vi "Dual_image_synced_snap_p_read_30psi.vi"() -> ()   [LabVIEW 2013]
uses:
  <vilib>/DAQmx/write.llb/DAQmx Write (Analog DBL 1Chan 1Samp).vi
  <vilib>/DAQmx/create/channels.llb/DAQmx Create Channel (AO-Voltage-Basic).vi
  <vilib>/DAQmx/create/channels.llb/DAQmx Create Channel (CO-Pulse Generation-Frequency).vi
  <vilib>/DAQmx/configure/timing.llb/DAQmx Timing (Implicit).vi
  <vilib>/DAQmx/miscellaneous.llb/DAQmx Fill In Error Info.vi
  <vilib>/vision/driver/NI_Vision_Acquisition_Software.lvlib
  <resource>/objmgr/imaqdx.rc
  <resource>/objmgr/daqmx.rc
panel:
  out "Snap Counter":u32
  in  "Snap":bool
  in  "Pressure Frequency (Hz)":dbl=10.0 format="%#_13g"
  in  "im num 2":string
  in  "im time 2":string
  out "im num":string
  out "im time":string
  out "Pressure Reading":cluster{dbl[], dbl[]}(graph)
  in  "Pressure Offset":dbl
  out "Current Pressure (Psi)":dbl format="%#.4g"
  in  "Gain 2":dbl(slide)=575.0 min=350.0 max=1000.0 step=1.0 scale=350.0..1000.0
  in  "VR2":dbl(slide)=65.0 min=0.0 max=255.0 step=1.0 scale=0.0..255.0
  in  "VR1":dbl(slide)=60.0 min=0.0 max=255.0 step=1.0 scale=0.0..255.0
  in  "UB2":dbl(slide)=160.0 min=0.0 max=255.0 step=1.0 scale=0.0..255.0
  in  "UB1":dbl(slide)=165.0 min=0.0 max=255.0 step=1.0 scale=0.0..255.0
  in  "Shutter":dbl(slide)=4095.0 min=0.0 max=4095.0 step=1.0 scale=4.095..4095.0 scale format="%#.0f"
  in  "Brightness":dbl(slide)=100.0 min=0.0 max=255.0 step=1.0 scale=0.0..255.0
  in  "Gain":dbl(slide)=600.0 min=350.0 max=1000.0 step=1.0 scale=350.0..1000.0
  in  "Test Description":string="test"
  in  "Storage Directory":path=path "C:/Users/Regen/Desktop/Users/Ryan Gergely/3D_DIC"
  out "Image 2":T1(plugin-control)
  out "Buffer Number 2":u32
  out "Frame Rate 2":dbl
  in  "Camera Name 2":refnum<k21>="cam2" caption="IMAQdx Session"
  in  "Image Frequency (Hz)":dbl=2.0 format="%.1f"
  out "Actual Duty Cycle":dbl
  out "Actual Frequency":dbl
  in  "Stop":bool
  in  "Start Trigger Mode":bool
  out "Frame Rate 1":dbl
  out "Buffer Number 1":u32
  in  "Camera Name 1":refnum<k21>="cam1" caption="IMAQdx Session"
  out "Image":T1(plugin-control)
  # "Exposure Settings - Both Cameras"
  # "White Balance - Camera1"
  # "White Balance - Camera2"
  # "1) Set Test Description and Storage Directory"
  # "2) Select Cameras"
  # "3) Start VI"
  # "4) Set Frequency and Exposure and White Balance\n(Before Start Trigger)"
  # "5)"
  # "6) Stop When Done"
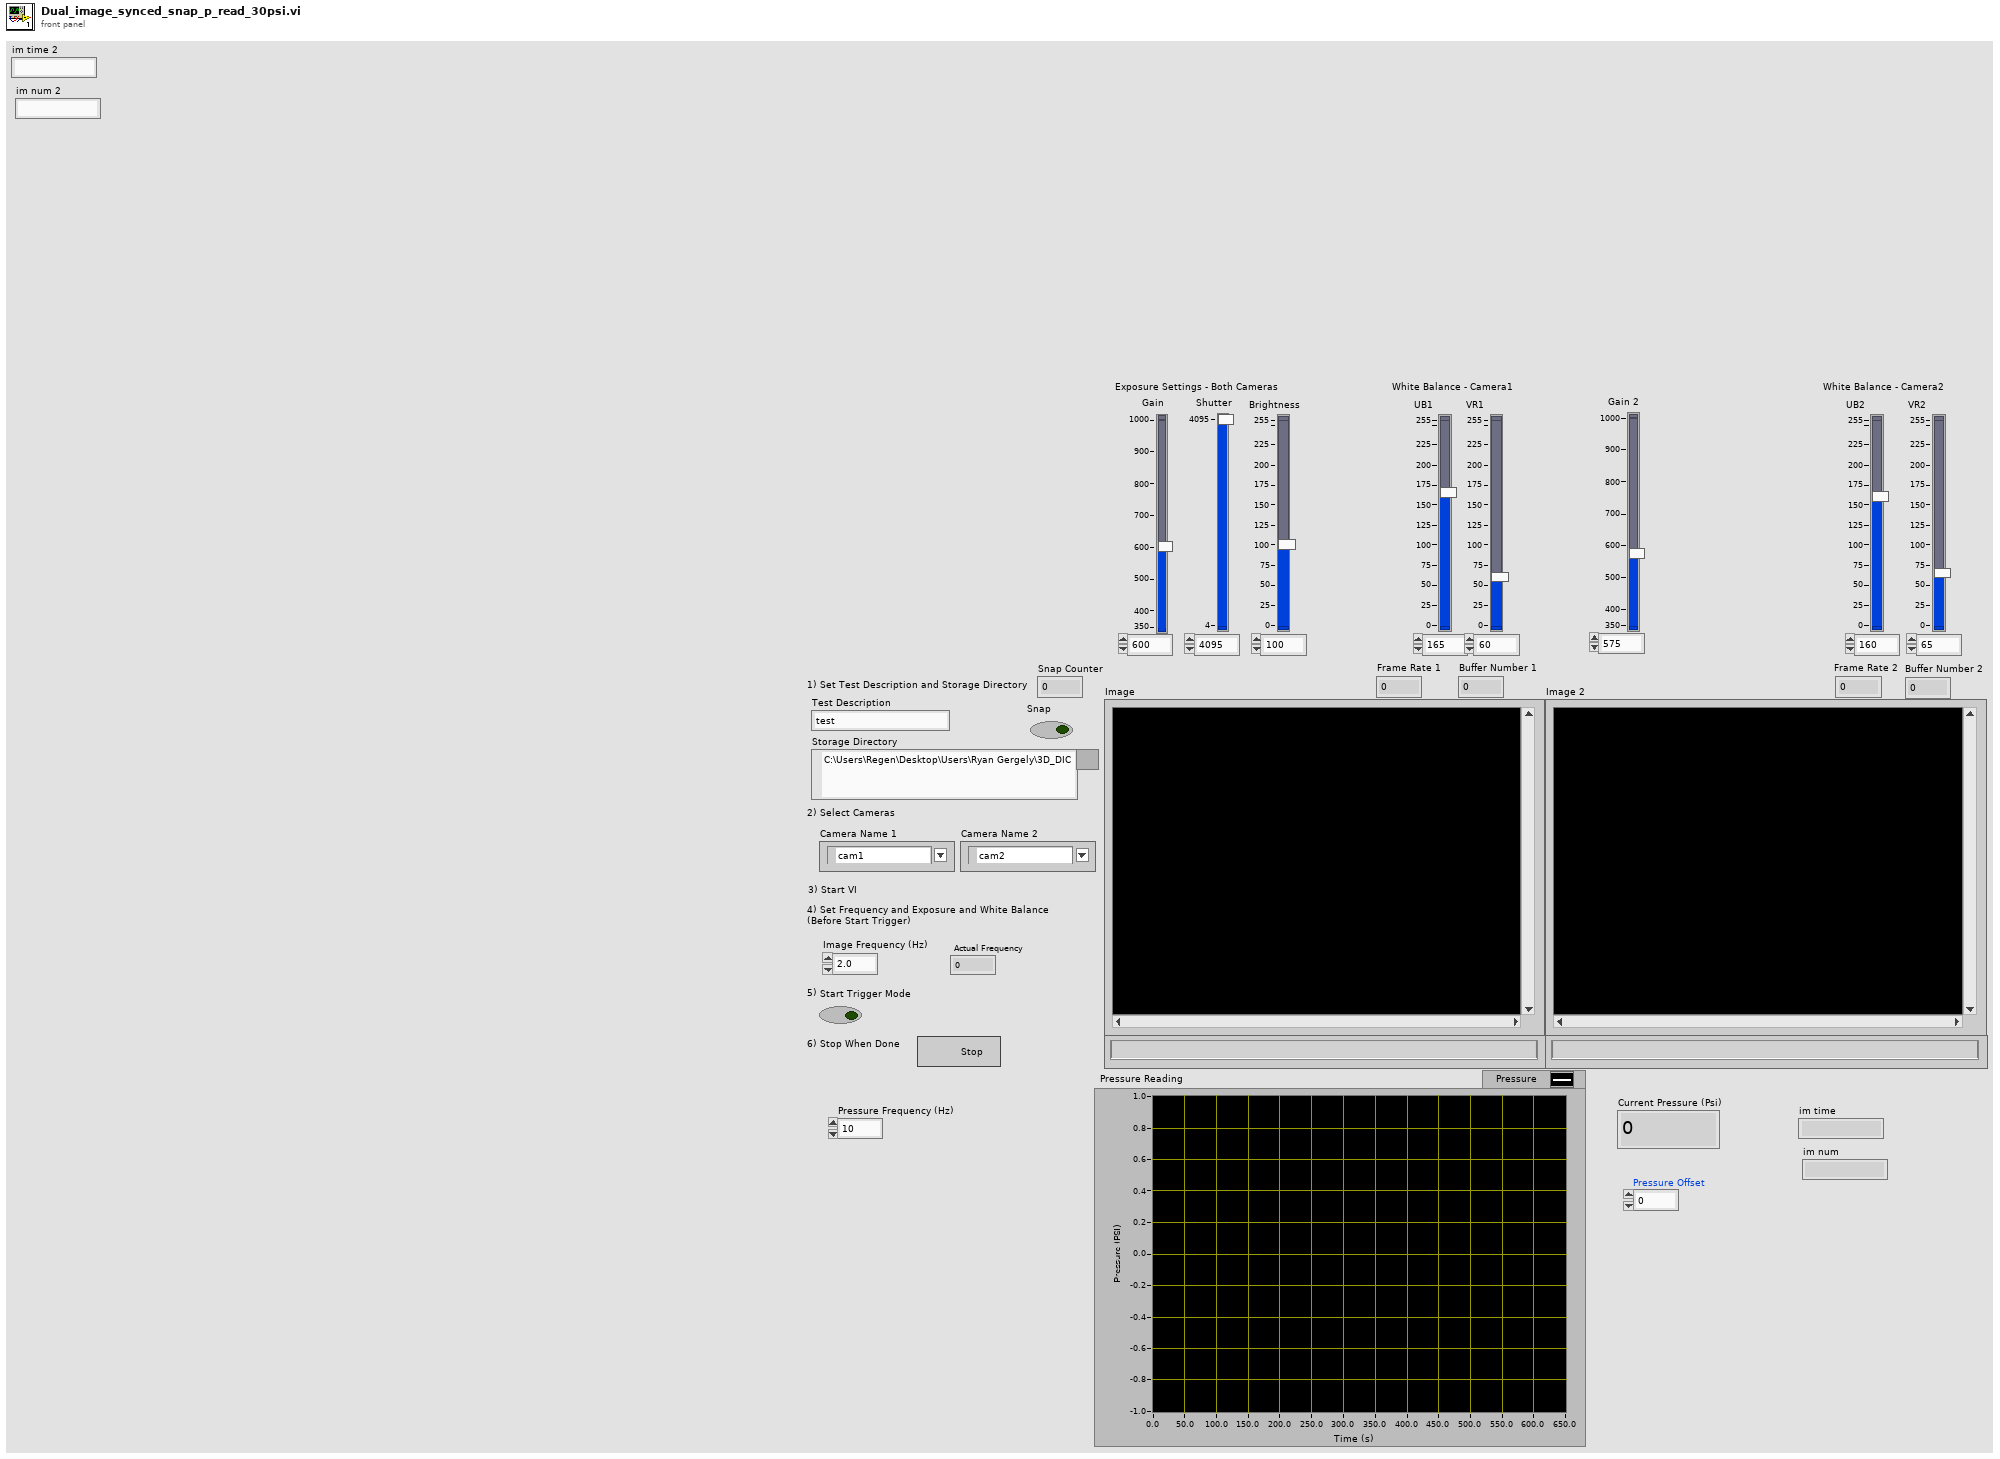
[diagram p1: front panel]
types:
  T1 = typedef "IMAQ Image.ctl" = refnum<image>
  T2 = enum16{"open", "open or create", "create or replace", "create", "open (read only)"}
  T3 = typedef "IMAQdx.ctl" = refnum<k21>
  T4 = enum16{"open", "replace", "create", "open or create", "replace or create", "replace or create with confirmation"}
  T5 = cluster{"Trigger Mode":u32, "Trigger Activation":u32, "Timeout (ms)":u32}
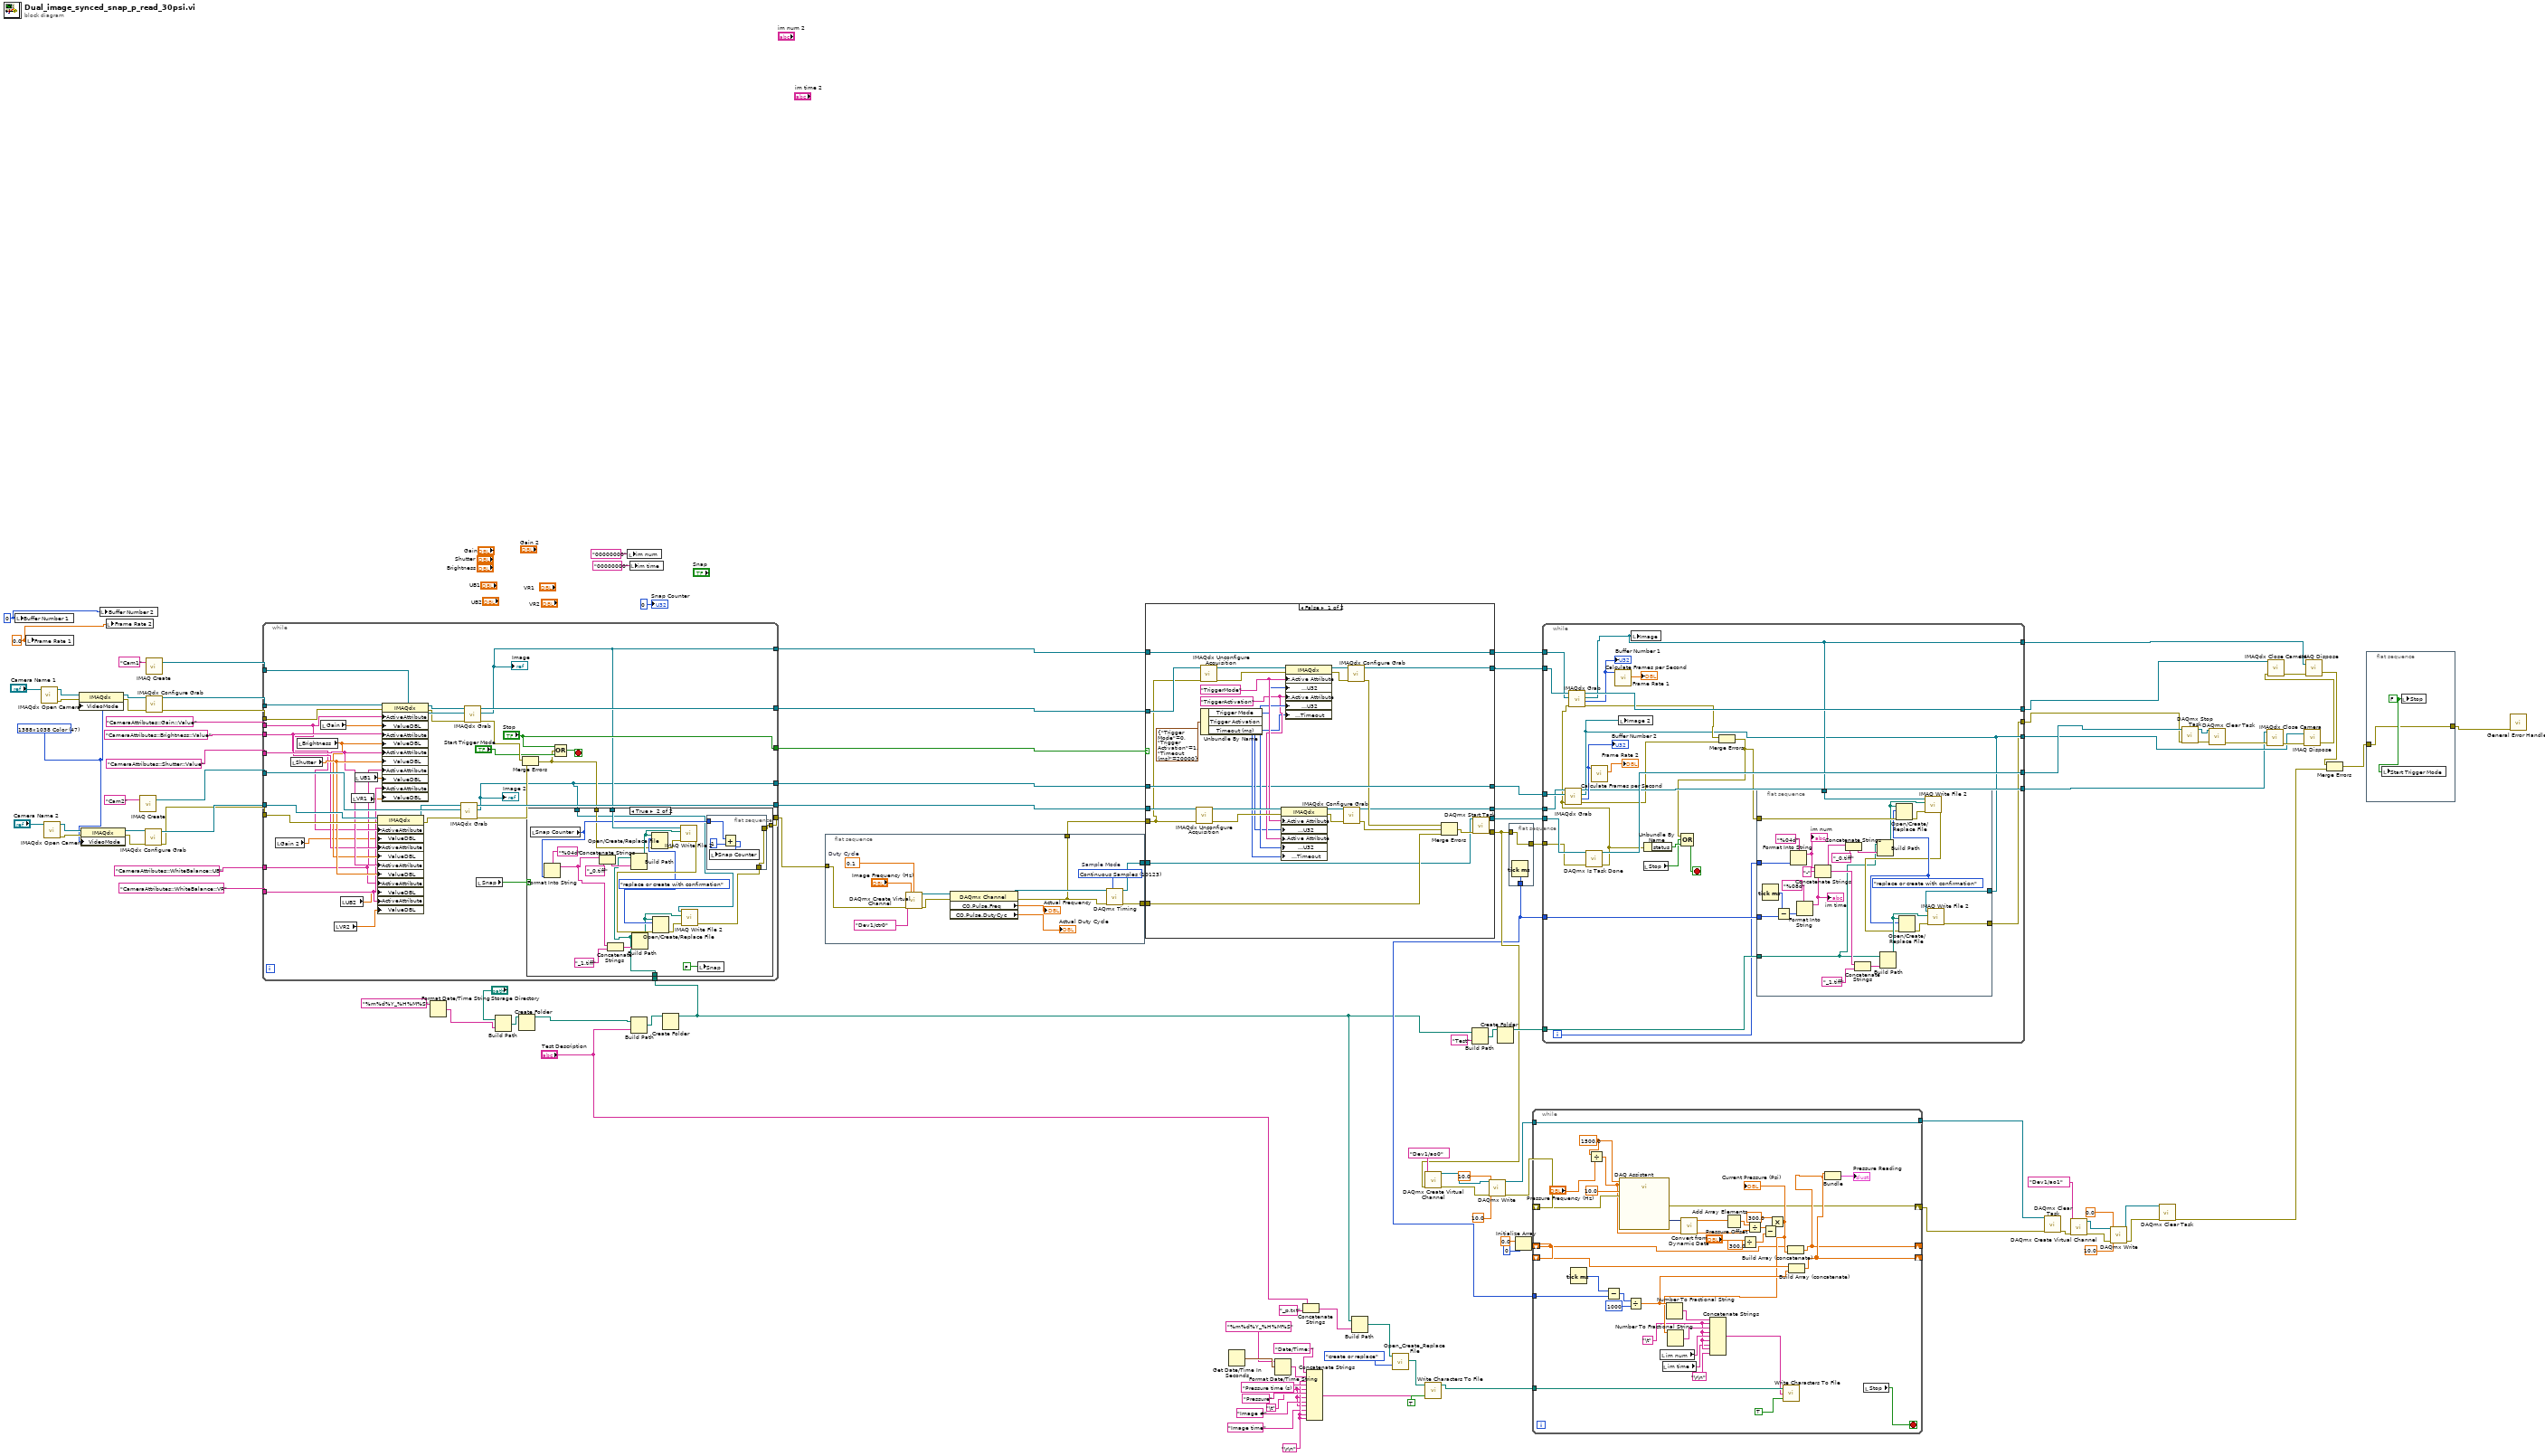
[diagram p0: block diagram]
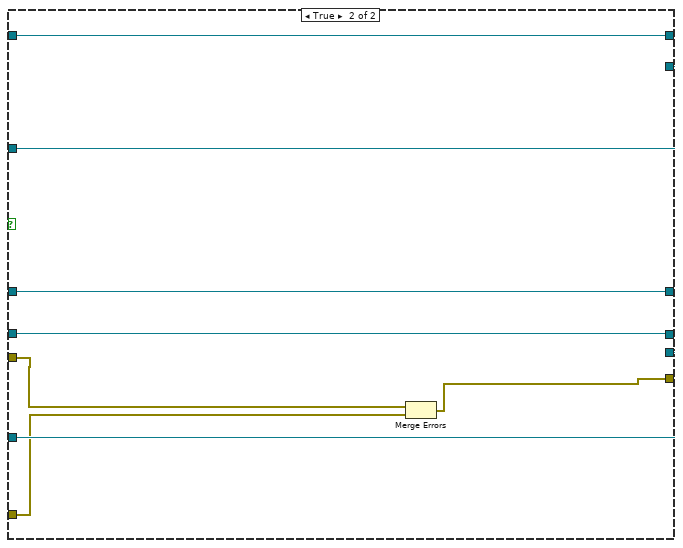
[diagram p2: hidden frame]
diagram:
  w2 = "\t"
  w4 = "\r\n"
  w61 = u32 47 items=["320x240 Color"=4, "640x480 Mono8"=9, "640x480 Mono16"=19, "640x480 Color"=14, "800x600 Mono8"=21, "800x600 Mono16"=27, "800x600 Color"=24, "1024x768 Mono8"=30, "1024x768 Mono16"=36, "1024x768 Color"=33, "1280x960 Mono8"=40, "1280x960 Mono16"=46, "1280x960 Color"=43, "1388x1038 Color"=47, "1388x1038 Mono"=48] ("Video Mode")
  w62 = 0.0 ("Frame Rate 1")
  w63 = u32 0 ("Buffer Number 1")
  n1 = local write "Buffer Number 1"(w63) -> ()
  n2 = local write "Frame Rate 1"(w62) -> ()
  n3 = call <vilib>:"IMAQdx Open Camera.vi"("Session In"="Camera Name 1") -> ("error out"=w69:errorcluster, "Session Out"=w71:T3)  [unwired: 2 in, 7 out]
  n4 = call <vilib>:"IMAQdx Open Camera.vi"("Session In"="Camera Name 2") -> ("error out"=w64:errorcluster, "Session Out"=w65:T3)  [unwired: 2 in, 7 out]
  n5 = property class="IMAQdx"(reference=w71, error in=w69, "VideoMode"=w61) -> (reference out=w70:T3, error out=w68:errorcluster)
  n6 = property class="IMAQdx"(reference=w65, error in=w64, "VideoMode"=w61) -> (reference out=w67:T3, error out=w66:errorcluster)
  n7 = local write "Buffer Number 2"(w63) -> ()
  n8 = local write "Frame Rate 2"(w62) -> ()
  n9 = call "IMAQ Create"("Image Name"="Cam2") -> ("New Image"=w58:T1)  [unwired: 3 in, 2 out]
  n10 = call <vilib>:"IMAQdx Configure Grab.vi"("error in"=w66, "Session In"=w67) -> ("error out"=w91:errorcluster, "Session Out"=w92:T3)  [unwired: 8 out]
  n11 = call "IMAQ Create"("Image Name"="Cam1") -> ("New Image"=w102:T1)  [unwired: 3 in, 2 out]
  n12 = call <vilib>:"IMAQdx Configure Grab.vi"("error in"=w68, "Session In"=w70) -> ("error out"=w100:errorcluster, "Session Out"=w101:T3)  [unwired: 8 out]
  n13 = Format Date/Time String(time format string (%c)="%m%d%Y_%H%M%S") -> (date/time string=w77:string)  [unwired: 2 in]
  n14 = Build Path(base path="Storage Directory", name or relative path=w77) -> (appended path=w79:path)
  n15 = Create Folder(path (use dialog)=w79) -> (created path=w27:path)  [unwired: 2 in, 2 out]
  n16 = local write "im num"("00000000" ("im num 2")) -> ()
  n17 = local write "im time"("00000000" ("im time 2")) -> ()
  n18 = Build Path(base path=w27, name or relative path="Test Description") -> (appended path=w75:path)
  n19 = Create Folder(path (use dialog)=w75) -> (created path=w6:path)  [unwired: 2 in, 2 out]
  n20 = while {
    tunnel: [w147] -> w109
    tunnel: w100 -> [w140]
    tunnel: w101 -> [w142]
    tunnel: w102 -> [w144]
    tunnel: [w116] -> w97
    tunnel: ["Stop"] -> w98
    tunnel: w92 -> [w138]
    tunnel: w91 -> [w137]
    tunnel: [w117] -> w60
    tunnel: [w145] -> w90
    tunnel: [w112] -> w89
    tunnel: w58 -> [w143]
    tunnel: "CameraAttributes::Shutter::Value" ("ActiveAttribute") -> [w133]
    tunnel: "CameraAttributes::Brightness::Value" ("ActiveAttribute") -> [w131]
    tunnel: "CameraAttributes::Gain::Value" ("ActiveAttribute") -> [w129]
    tunnel: "CameraAttributes::WhiteBalance::UB" ("ActiveAttribute") -> [w126]
    tunnel: "CameraAttributes::WhiteBalance::VR" ("ActiveAttribute") -> [w127]
    tunnel: w6 -> [w114]
    stop <- w121 stop-if-true
    n21 = local read "Gain 2"() -> (w122:dbl)
    n22 = local read "Shutter"() -> (w134:dbl)
    n23 = local read "Brightness"() -> (w132:dbl)
    n24 = local read "Gain"() -> (w130:dbl)
    n25 = local read "VR2"() -> (w123:dbl)
    n26 = local read "UB2"() -> (w125:dbl)
    n27 = local read "VR1"() -> (w124:dbl)
    n28 = local read "UB1"() -> (w128:dbl)
    n29 = property class="IMAQdx"(reference=w138, error in=w137, "ActiveAttribute"=w129, "ValueDBL"=w122, "ActiveAttribute"=w131, "ValueDBL"=w132, "ActiveAttribute"=w133, "ValueDBL"=w134, "ActiveAttribute"=w126, "ValueDBL"=w125, "ActiveAttribute"=w127, "ValueDBL"=w123) -> (reference out=w135:T3, error out=w136:errorcluster)
    n30 = property class="IMAQdx"(reference=w142, error in=w140, "ActiveAttribute"=w129, "ValueDBL"=w130, "ActiveAttribute"=w131, "ValueDBL"=w132, "ActiveAttribute"=w133, "ValueDBL"=w134, "ActiveAttribute"=w126, "ValueDBL"=w128, "ActiveAttribute"=w127, "ValueDBL"=w124) -> (reference out=w141:T3, error out=w139:errorcluster)
    n31 = call <vilib>:"IMAQdx Grab.vi"("error in"=w136, "Image In"=w143, "Session In"=w135) -> ("error out"=w118:errorcluster, "Image Out"=w112:T1, "Session Out"=w145:T3)  [unwired: 1 in, 5 out]
    "Image 2" <- w112
    n32 = call <vilib>:"IMAQdx Grab.vi"("error in"=w139, "Image In"=w144, "Session In"=w141) -> ("error out"=w120:errorcluster, "Image Out"=w116:T1, "Session Out"=w147:T3)  [unwired: 1 in, 5 out]
    "Image" <- w116
    n33 = local read "Snap"() -> (w113:bool)
    n34 = Merge Errors(w120, w118) -> (w115:errorcluster)
    n35 = case shown="True" w113 {
      tunnel: [w148 w153] -> w117
      tunnel: w116 -> [_ w157]
      tunnel: w114 -> [_ w151]
      tunnel: w115 -> [w148 w150]
      tunnel: w112 -> [_ w149]
      frame False {
      }
      frame True {
        w160 = T4."replace or create with confirmation" ("operation (0:open)")
        n36 = local read "Snap Counter"() -> (w155:u32)
        n37 = Format Into String(format string="%04d", w155) -> (resulting string=w152:string)  [unwired: 2 in, 1 out]
        n38 = Concatenate Strings(w152, "_0.tiff") -> (w165:string)
        n39 = Concatenate Strings(w152, "_1.tiff") -> (w164:string)
        n40 = Build Path(base path=w151, name or relative path=w165) -> (appended path=w158:path)
        n41 = Build Path(base path=w151, name or relative path=w164) -> (appended path=w159:path)
        n42 = Open/Create/Replace File(file path (use dialog)=w158, error in=w150, operation (0:open)=w160) -> (error out=w161:errorcluster)  [unwired: 3 in, 2 out]
        n43 = call-poly "IMAQ Write File 2"("error in (no error)"=w161, "File Path"=w158, "Image"=w157) -> ("error out"=w163:errorcluster)  [unwired: 7 in, 1 out]
        n44 = Open/Create/Replace File(file path (use dialog)=w159, error in=w163, operation (0:open)=w160) -> (error out=w162:errorcluster)  [unwired: 3 in, 2 out]
        n45 = call-poly "IMAQ Write File 2"("error in (no error)"=w162, "File Path"=w159, "Image"=w149) -> ("error out"=w154:errorcluster)  [unwired: 7 in, 1 out]
        n46 = local write "Snap"(FALSE ("Ready?")) -> ()
        n47 = flat-sequence {
          tunnel: w155 -> [w172]
          tunnel: w154 -> [w169]
          tunnel: [w169] -> w153
          frame #0 {
            n48 = Add(x=w172, y=u32 1) -> (x+y=w170:u32)
            n49 = local write "Snap Counter"(w170) -> ()
          }
        }
      }
    }
    n50 = Compound Arithmetic op=OR("Stop", w115, "Start Trigger Mode") -> (w121:bool)
  }
  n51 = flat-sequence {
    tunnel: [w176] -> w95
    tunnel: [w175] -> w88
    tunnel: w60 -> [w174]
    tunnel: [w173] -> w59
    frame #0 {
      w183 = 0.1  # Duty Cycle
      w177 = 10123 items=["Finite Samples"=10178, "Continuous Samples"=10123, "Hardware Timed Single Point"=12522]  # Sample Mode
      n52 = call-poly <vilib>:"DAQmx Create Virtual Channel.vi"("frequency"="Image Frequency (Hz)", "duty cycle"=w183, "counter"=tag "Dev1/ctr0" ("Counter"), "error in"=w174) -> ("task out"=w179:refnum<k21>, "error out"=w180:errorcluster)  [unwired: 10 in]
      n53 = property class="DAQmx Channel"(reference=w179, error in=w180) -> (reference out=w181:refnum<k21>, error out=w173:errorcluster, "CO.Pulse.Freq"=→"Actual Frequency":dbl, "CO.Pulse.DutyCyc"=→"Actual Duty Cycle":dbl)
      n54 = call-poly <vilib>:"DAQmx Timing.vi"("task/channels in"=w181, "sample mode"=w177, "error in"=w173) -> ("task out"=w176:refnum<k21>, "error out"=w175:errorcluster)  [unwired: 11 in]
    }
  }
  n55 = case shown="False" w98 {
    tunnel: w109 -> [w213 w221]
    tunnel: [w212 w221] -> w108
    tunnel: [w194 w214] -> w16
    tunnel: [w195 w219] -> w106
    tunnel: w97 -> [w206 w220]
    tunnel: [w206 w220] -> w96
    tunnel: w95 -> [w187 w219]
    tunnel: w59 -> [w186 w218]
    tunnel: w90 -> [w197 w215]
    tunnel: w89 -> [w196 w216]
    tunnel: [w196 w216] -> w87
    tunnel: w88 -> [w190 w217]
    tunnel: [w188 w215] -> w86
    frame False {
      w200 = "TriggerActivation" ("ActiveAttribute")
      w202 = "TriggerMode" ("ActiveAttribute")
      n56 = call <vilib>:"IMAQdx Unconfigure Acquisition.vi"("error in"=w186, "Session In"=w197) -> ("error out"=w204:errorcluster, "Session Out"=w203:T3)  [unwired: 8 out]
      n57 = call <vilib>:"IMAQdx Unconfigure Acquisition.vi"("error in"=w186, "Session In"=w213) -> ("error out"=w209:errorcluster, "Session Out"=w208:T3)  [unwired: 8 out]
      n58 = Unbundle By Name(T5 {"Trigger Mode"=0, "Trigger Activation"=1, "Timeout (ms)"=20000} ("Trigger Parameters")) -> ("Trigger Mode"=w198:u32, "Trigger Activation"=w201:u32, "Timeout (ms)"=w199:u32)
      n59 = property class="IMAQdx"(reference=w203, error in=w204, "Camera Attributes:Active Attribute"=w202, "Camera Attributes:Value:U32"=w198, "Camera Attributes:Active Attribute"=w200, "Camera Attributes:Value:U32"=w201, "Acquisition Attributes:Timeout"=w199) -> (reference out=w205:T3, error out=w193:errorcluster)
      n60 = property class="IMAQdx"(reference=w208, error in=w209, "Camera Attributes:Active Attribute"=w202, "Camera Attributes:Value:U32"=w198, "Camera Attributes:Active Attribute"=w200, "Camera Attributes:Value:U32"=w201, "Acquisition Attributes:Timeout"=w199) -> (reference out=w210:T3, error out=w211:errorcluster)
      n61 = call <vilib>:"IMAQdx Configure Grab.vi"("error in"=w193, "Session In"=w205) -> ("error out"=w191:errorcluster, "Session Out"=w188:T3)  [unwired: 8 out]
      n62 = call <vilib>:"IMAQdx Configure Grab.vi"("error in"=w211, "Session In"=w210) -> ("error out"=w189:errorcluster, "Session Out"=w212:T3)  [unwired: 8 out]
      n63 = Merge Errors(w189, w191, w190) -> (w192:errorcluster)
      n64 = call <vilib>:"DAQmx Start Task.vi"("task/channels in"=w187, "error in"=w192) -> ("task out"=w195:refnum<k21>, "error out"=w194:errorcluster)  [unwired: 12 in]
    }
    frame True {
      n65 = Merge Errors(w218, w217) -> (w214:errorcluster)
    }
  }
  n66 = Get Date/Time In Seconds() -> (seconds since 1Jan1904=w39:timestamp)
  n67 = Format Date/Time String(time format string (%c)="%m%d%Y_%H%M%S", seconds (now)=w39) -> (date/time string=w45:string)  [unwired: 1 in]
  n68 = Concatenate Strings("Test Description", "_p.txt" ("string")) -> (w50:string)
  n69 = Concatenate Strings("Date/Time: ", w45, w4, "Pressure time (s)  ", w2, "Pressure" ("string"), w2, "Image #" ("string"), w2, "Image time" ("string"), w4, w4) -> (w46:string)
  n70 = Build Path(base path=w6, name or relative path=w50) -> (appended path=w42:path)
  n71 = call <vilib>:"Open_Create_Replace File.vi"("function (open:0)"=T2."create or replace", "file path"=w42) -> ("new file path"=w48:path)  [unwired: 6 in, 3 out]
  n72 = call-poly <vilib>:"DAQmx Create Virtual Channel.vi"("physical channels"=tag "Dev1/ao0", "error in"=w16) -> ("task out"=w30:refnum<k21>, "error out"=w34:errorcluster)  [unwired: 12 in]
  n73 = call <vilib>:"Write Characters To File.vi"("append to file? (new file:F)"=TRUE, "character string"=w46, "file path (dialog if empty)"=w48) -> ("new file path (Not A Path if cancelled)"=w41:path)  [unwired: 2 in]
  n74 = Build Path(base path=w6, name or relative path="Test") -> (appended path=w73:path)
  n75 = call-poly <vilib>:"DAQmx Write.vi"("task/channels in"=w30, "data"=10.0, "timeout"=10.0, "error in"=w34) -> ("task out"=w28:refnum<k21>, "error out"=w29:errorcluster)  [unwired: 9 in, 1 out]
  n76 = Create Folder(path (use dialog)=w73) -> (created path=w72:path)  [unwired: 2 in, 2 out]
  n77 = flat-sequence {
    tunnel: w16 -> [w223]
    tunnel: [w223] -> w52
    tunnel: [w222] -> w15
    frame #0 {
      n78 = Tick Count (ms)() -> (millisecond timer value=w222:u32)
    }
  }
  n79 = Initialize Array(0.0 ("element"), 0 ("dimension size")) -> (w36:dbl[])
  n80 = while {
    tunnel: w41 -> [w260]
    tunnel: w15 -> [w257]
    shift-right: [w235] -> w5
    shift-left: w29 -> [w250]
    shift-right: [w242] -> _
    shift-left: w36 -> [w236]
    shift-right: [w243] -> _
    shift-left: w36 -> [w245]
    tunnel: w28 -> [w241]
    tunnel: [w241] -> w18
    stop <- w225 stop-if-true
    w231 = 1500.0 ("rate")
    w228 = "\t"
    n81 = Tick Count (ms)() -> (millisecond timer value=w258:u32)
    n82 = Divide(x=w231, y="Pressure Frequency (Hz)") -> (x/y=w230:dbl)
    n83 = Subtract(x=w258, y=w257) -> (x-y=w256:u32)
    n84 = call "DAQ Assistant"("rate"=w231, "number of samples"=w230, "timeout (s)"=10.0, "error in"=w250) -> ("data"=w251:dynamicdata, "error out"=w235:errorcluster)  [unwired: 13 in, 1 out]
    n85 = Divide(x=w256, y=u32 1000) -> (x/y=w246:dbl)
    n86 = local read "im num"() -> (w229:string)
    n87 = local read "im time"() -> (w227:string)
    n88 = Number To Fractional String(number=w246) -> (F-format string=w254:string)  [unwired: 3 in]
    n89 = call "Convert from Dynamic Data"("Dynamic Data Type"=w251) -> ("Array"=w248:dbl[])  [unwired: 3 in]
    n90 = Add Array Elements(numeric array=w248) -> (sum=w247:dbl)
    n91 = Divide(x="Pressure Offset", y=300.0) -> (x/y=w232:dbl)
    n92 = Divide(x=w247, y=w230) -> (x/y=w240:dbl)
    n93 = Subtract(x=w240, y=w232) -> (x-y=w238:dbl)
    n94 = Multiply(x=w238, y=300.0) -> (x*y=w237:dbl)
    "Current Pressure (Psi)" <- w237
    n95 = Number To Fractional String(number=w237) -> (F-format string=w253:string)  [unwired: 3 in]
    n96 = Concatenate Strings(w254, w228, w253, w228, w229, w228, w227, w228, "\r\n") -> (w252:string)
    n97 = call <vilib>:"Write Characters To File.vi"("append to file? (new file:F)"=TRUE, "character string"=w252, "file path (dialog if empty)"=w260) -> ()  [unwired: 2 in, 1 out]
    n98 = Build Array (concatenate)(w236, w237) -> (w242:dbl[])
    n99 = Build Array (concatenate)(w245, w246) -> (w243:dbl[])
    n100 = Bundle(w243, w242) -> (→"Pressure Reading":cluster{dbl[], dbl[]})  [unwired: 1 in]
    n101 = local read "Stop"() -> (w225:bool)
  }
  n102 = while {
    tunnel: [w286] -> w104
    tunnel: [w264] -> w10
    tunnel: w108 -> [w283]
    tunnel: w96 -> [w282]
    tunnel: [w279] -> w103
    tunnel: w106 -> [w278]
    tunnel: w87 -> [w275]
    tunnel: w86 -> [w274]
    tunnel: w52 -> [w271]
    tunnel: [w268] -> w80
    tunnel: [w267] -> w82
    tunnel: [w270] -> w81
    tunnel: w72 -> [w269]
    tunnel: w15 -> [w263]
    i -> [w261]
    stop <- w280 stop-if-true
    n103 = call <vilib>:"DAQmx Is Task Done.vi"("task/channels in"=w278, "error in"=w271) -> ("task out"=w279:refnum<k21>, "error out"=w265:errorcluster)  [unwired: 11 in, 1 out]
    n104 = call <vilib>:"IMAQdx Grab.vi"("error in"=w265, "Image In"=w275, "Session In"=w274) -> ("error out"=w266:errorcluster, "Buffer Number Out"=w273:u32, "Image Out"=w267:T1, "Session Out"=w270:T3)  [unwired: 1 in, 4 out]
    "Buffer Number 2" <- w273
    n105 = call <vilib>:"IMAQdx Grab.vi"("error in"=w265, "Image In"=w282, "Session In"=w283) -> ("error out"=w272:errorcluster, "Buffer Number Out"=w284:u32, "Image Out"=w268:T1, "Session Out"=w286:T3)  [unwired: 1 in, 4 out]
    "Buffer Number 1" <- w284
    n106 = call <vilib>:"Calculate Frames per Second.vi"("Buffer Number"=w273) -> ("Processed Frames/s"=→"Frame Rate 2":dbl)  [unwired: 8 in, 2 out]
    n107 = call <vilib>:"Calculate Frames per Second.vi"("Buffer Number"=w284) -> ("Processed Frames/s"=→"Frame Rate 1":dbl)  [unwired: 8 in, 2 out]
    n108 = local write "Image 2"(w267) -> ()
    n109 = local write "Image"(w268) -> ()
    n110 = Unbundle By Name(w265) -> ("status"=w281:bool)
    n111 = local read "Stop"() -> (w277:bool)
    n112 = Merge Errors(w272, w266) -> (w262:errorcluster)
    n113 = Compound Arithmetic op=OR(w262, w277, w281) -> (w280:bool)
    n114 = flat-sequence {
      tunnel: w269 -> [w287]
      tunnel: w268 -> [w311]
      tunnel: w267 -> [w310]
      tunnel: w262 -> [w309]
      tunnel: [w308] -> w264
      tunnel: w263 -> [w301]
      tunnel: w261 -> [w293]
      frame #0 {
        w305 = T4."replace or create with confirmation" ("operation (0:open)")
        n115 = Tick Count (ms)() -> (millisecond timer value=w300:u32)
        n116 = Subtract(x=w300, y=w301) -> (x-y=w296:u32)
        n117 = Format Into String(format string="%04d", w293) -> (resulting string=w291:string)  [unwired: 2 in, 1 out]
        "im num" <- w291
        n118 = Format Into String(format string="%08d", w296) -> (resulting string=w295:string)  [unwired: 2 in, 1 out]
        "im time" <- w295
        n119 = Concatenate Strings(w291, "-" ("string"), w295) -> (w288:string)
        n120 = Concatenate Strings(w288, "_0.tiff") -> (w298:string)
        n121 = Concatenate Strings(w288, "_1.tiff") -> (w299:string)
        n122 = Build Path(base path=w287, name or relative path=w298) -> (appended path=w307:path)
        n123 = Build Path(base path=w287, name or relative path=w299) -> (appended path=w306:path)
        n124 = Open/Create/Replace File(file path (use dialog)=w307, error in=w309, operation (0:open)=w305) -> (error out=w304:errorcluster)  [unwired: 3 in, 2 out]
        n125 = call-poly "IMAQ Write File 2"("error in (no error)"=w304, "File Path"=w307, "Image"=w311) -> ("error out"=w302:errorcluster)  [unwired: 7 in, 1 out]
        n126 = Open/Create/Replace File(file path (use dialog)=w306, error in=w302, operation (0:open)=w305) -> (error out=w303:errorcluster)  [unwired: 3 in, 2 out]
        n127 = call-poly "IMAQ Write File 2"("error in (no error)"=w303, "File Path"=w306, "Image"=w310) -> ("error out"=w308:errorcluster)  [unwired: 7 in, 1 out]
      }
    }
  }
  n128 = call <vilib>:"DAQmx Clear Task.vi"("task in"=w18, "error in"=w5) -> ("error out"=w25:errorcluster)  [unwired: 13 in]
  n129 = call-poly <vilib>:"DAQmx Create Virtual Channel.vi"("physical channels"=tag "Dev1/ao1", "error in"=w25) -> ("task out"=w20:refnum<k21>, "error out"=w26:errorcluster)  [unwired: 12 in]
  n130 = call-poly <vilib>:"DAQmx Write.vi"("task/channels in"=w20, "data"=0.0, "timeout"=10.0, "error in"=w26) -> ("task out"=w19:refnum<k21>, "error out"=w24:errorcluster)  [unwired: 9 in, 1 out]
  n131 = call <vilib>:"DAQmx Clear Task.vi"("task in"=w19, "error in"=w24) -> ("error out"=w13:errorcluster)  [unwired: 13 in]
  n132 = call <vilib>:"DAQmx Stop Task.vi"("task/channels in"=w103, "error in"=w10) -> ("task out"=w105:refnum<k21>, "error out"=w107:errorcluster)  [unwired: 12 in]
  n133 = call <vilib>:"DAQmx Clear Task.vi"("task in"=w105, "error in"=w107) -> ("error out"=w83:errorcluster)  [unwired: 13 in]
  n134 = call <vilib>:"IMAQdx Close Camera.vi"("error in"=w83, "Session In"=w81) -> ("error out"=w85:errorcluster)  [unwired: 9 out]
  n135 = call "IMAQ Dispose"("Image"=w82, "error in (no error)"=w85) -> ("error out"=w84:errorcluster)  [unwired: 4 in]
  n136 = call <vilib>:"IMAQdx Close Camera.vi"("error in"=w84, "Session In"=w104) -> ("error out"=w111:errorcluster)  [unwired: 9 out]
  n137 = call "IMAQ Dispose"("Image"=w80, "error in (no error)"=w111) -> ("error out"=w14:errorcluster)  [unwired: 4 in]
  n138 = Merge Errors(w14, w13) -> (w9:errorcluster)
  n139 = flat-sequence {
    tunnel: w9 -> [w312]
    tunnel: [w312] -> w8
    frame #0 {
      w313 = FALSE ("Stop")
      n140 = local write "Start Trigger Mode"(w313) -> ()
      n141 = local write "Stop"(w313) -> ()
    }
  }
  n142 = call <vilib>:"General Error Handler.vi"("error in (no error)"=w8) -> ()  [unwired: 1 in, 14 out]
  "Snap Counter" <- u32 0 ("Snap Counter")
